vi "Save Load.vi"(6 "error in":errorcluster, 7 "save/load cluster":T3={"OK Button"=FALSE, "OK Button 2"=FALSE, "OK Button 3"=TRUE, "OK Button 4"=FALSE}, 11 "home path":path=path "C:/control") -> (4 "error out 3":errorcluster)   [LabVIEW 2016, in "Save Load.lvlib"]
doc: "Takes a vi and saves or loads set values depending on which cluster value is chosen"
uses:
  Save Load.lvlib
  Users/wymanm/Desktop/Control computer - Copy/control/control vi/ion Source/Ion Source/ion source llb.lvlib
  save or load.ctl
  all or current.ctl
  file or temp.ctl
  Users/wymanm/Desktop/Control computer - Copy/control/control vi/main/save load/saveload.ctl
  main.lvlib
  save load method.ctl
  beamline selection.ctl
panel:
  in  "Beamline Section":T1
  in  "Save Load Method":T2
  out "appended array":string[](array[string])
  out "path":path
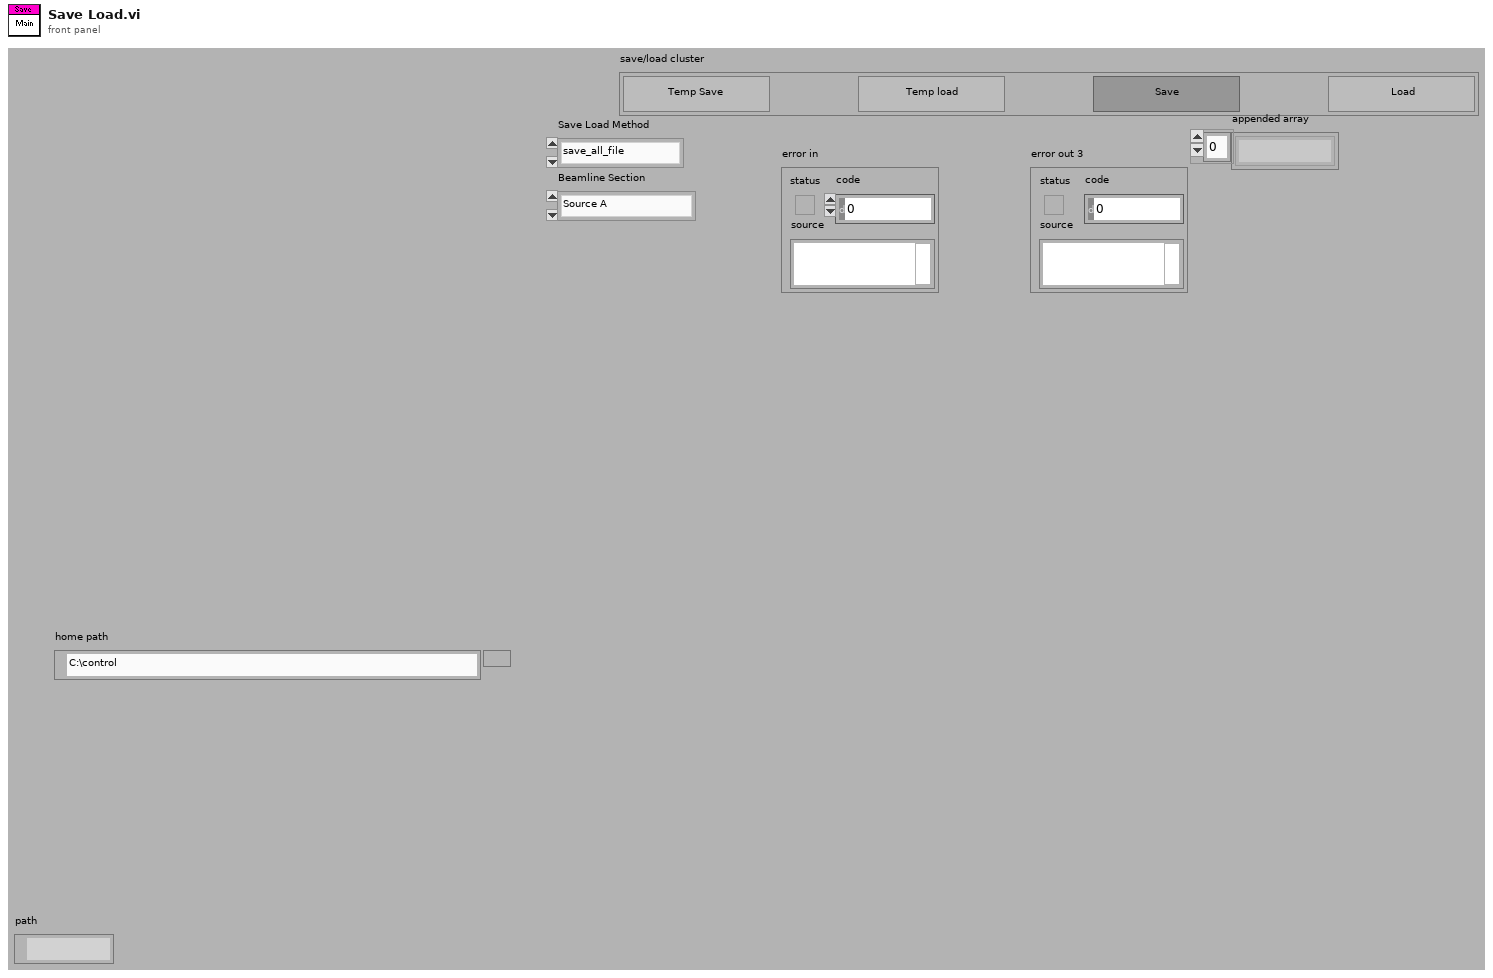
[diagram p1: front panel]
types:
  T1 = typedef "main.lvlib/beamline selection.ctl" = enum16{"Source A", "Source B", "Low Energy End", "High Energy End", "Transmission", "R30", "R45"}
  T2 = typedef "Save Load.lvlib/save load method.ctl" = enum16{"save_all_file", "save_all_temp", "save_curr_file", "save_curr_temp", "load_all_file", "load_all_temp", "load_curr_file", "load_curr_temp"}
  T3 = typedef "main.lvlib/saveload.ctl" = cluster{"OK Button":bool, "OK Button 2":bool, "OK Button 3":bool, "OK Button 4":bool}
  T4 = enum16{"open", "replace", "create", "open or create", "replace or create", "replace or create with confirmation"}
  T5 = typedef "file or temp.ctl" = enum16{"file", "temp"}
  T6 = typedef "all or current.ctl" = enum16{"current", "all"}
  T7 = typedef "save or load.ctl" = enum16{"save", "load"}
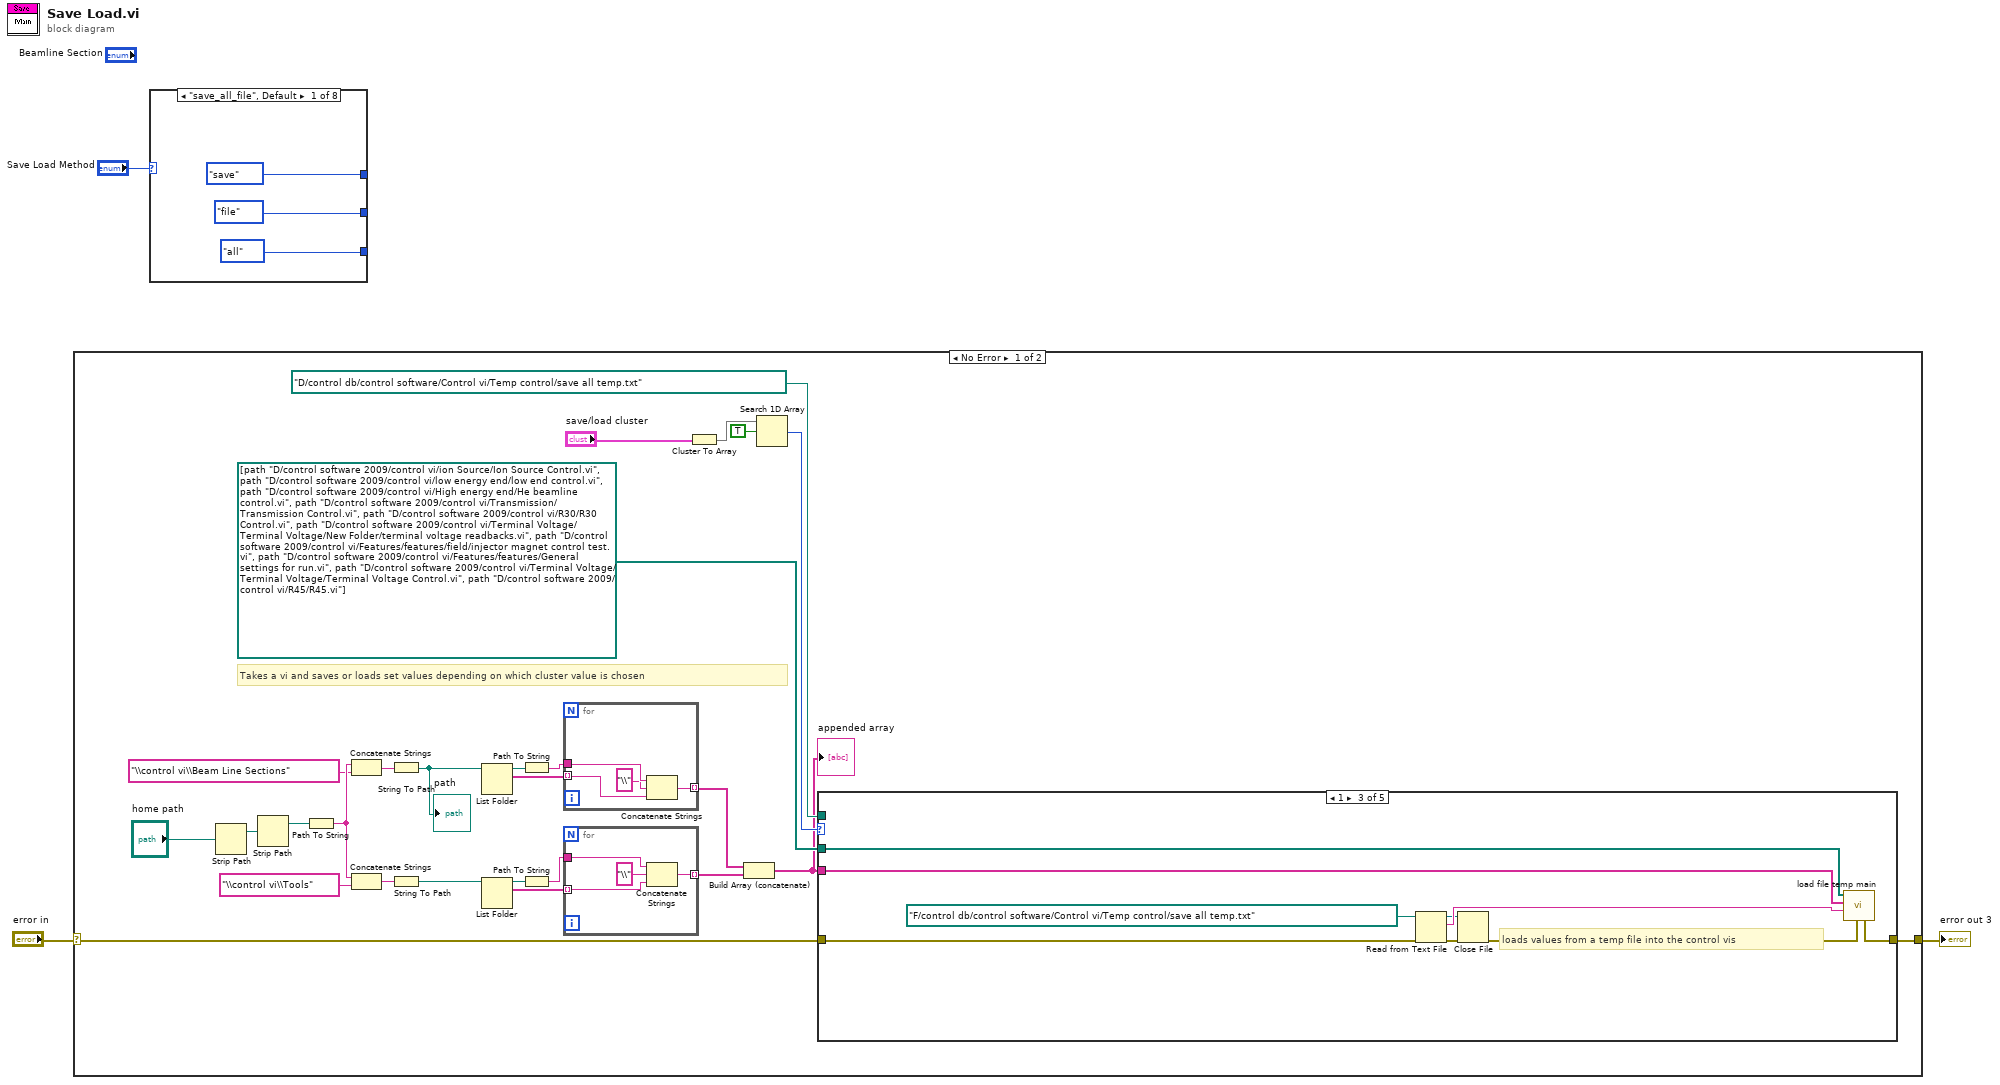
[diagram p0: block diagram]
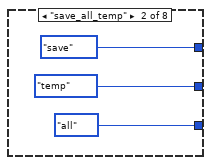
[diagram p2: hidden frame]
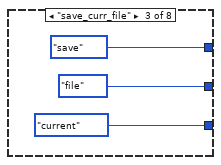
[diagram p3: hidden frame]
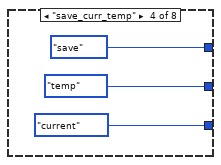
[diagram p4: hidden frame]
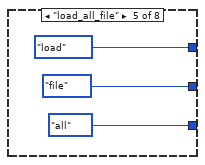
[diagram p5: hidden frame]
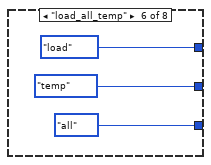
[diagram p6: hidden frame]
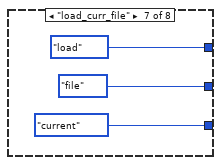
[diagram p7: hidden frame]
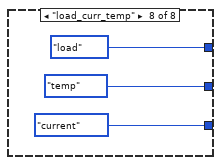
[diagram p8: hidden frame]
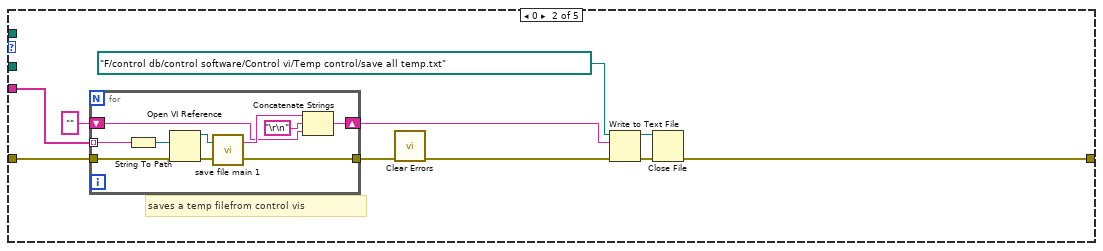
[diagram p10: hidden frame]
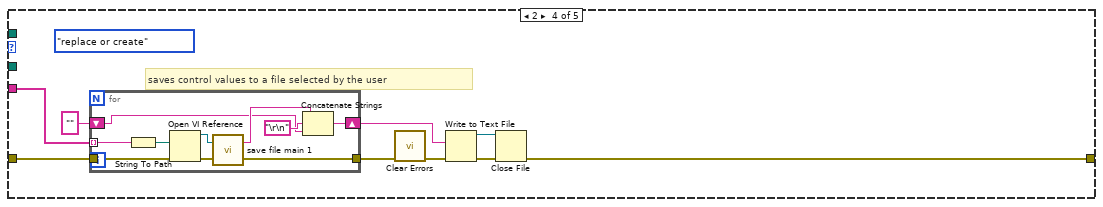
[diagram p11: hidden frame]
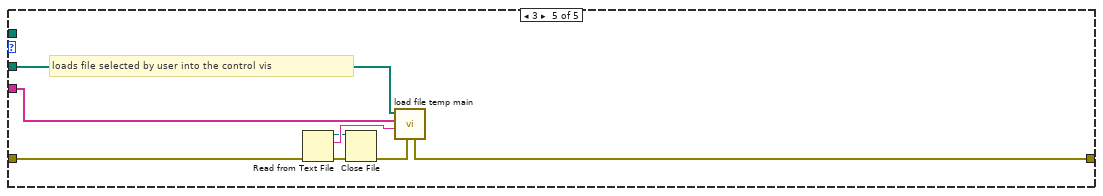
[diagram p12: hidden frame]
diagram:
  n1 = case shown="No Error" "error in" {
    selector: "error in" -> [w24 w96]
    tunnel: [w25 w96] -> w3
    frame No Error {
      # "Takes a vi and saves or loads set values depending on which cluster value is chosen"
      n2 = Strip Path(path="home path") -> (stripped path=w5:path)  [unwired: 1 out]
      n3 = Strip Path(path=w5) -> (stripped path=w4:path)  [unwired: 1 out]
      n4 = Path To String(path=w4) -> (string=w13:string)
      n5 = Concatenate Strings(w13, "\\control vi\\Beam Line Sections" ("string")) -> (w11:string)
      n6 = Concatenate Strings(w13, "\\control vi\\Tools" ("string")) -> (w14:string)
      n7 = String To Path(string=w11) -> (path=w12:path)
      "path" <- w12
      n8 = String To Path(string=w14) -> (path=w15:path)
      n9 = List Folder(path=w12) -> (path out=w21:path, filenames=w20:string[])  [unwired: 3 in, 2 out]
      n10 = List Folder(path=w15) -> (path out=w16:path, filenames=w18:string[])  [unwired: 3 in, 2 out]
      n11 = Path To String(path=w21) -> (string=w19:string)
      n12 = Path To String(path=w16) -> (string=w17:string)
      n13 = for {
        tunnel: w19 -> [w34]
        tunnel: w20 -> [w32] mode=indexing
        tunnel: [w31] -> w22 mode=indexing
        n14 = Concatenate Strings(w34, "\\" ("string"), w32) -> (w31:string)
      }
      n15 = for {
        tunnel: w17 -> [w38]
        tunnel: w18 -> [w36] mode=indexing
        tunnel: [w35] -> w23 mode=indexing
        n16 = Concatenate Strings(w38, "\\" ("string"), w36) -> (w35:string)
      }
      n17 = Cluster To Array(cluster="save/load cluster") -> (array=w29:bool[])
      n18 = Build Array (concatenate)(w22, w23) -> (w7:string[])
      "appended array" <- w7
      n19 = Search 1D Array(1D array=w29, element=TRUE) -> (index of element=w27:i32)  [unwired: 1 out]
      n20 = case shown="1" w27 {
        tunnel: path "D:/control db/control software/Control vi/Temp control/save all temp.txt" ("file path (use dialog)") -> [_ _ _ _ _]
        tunnel: path[] [path "D:/control software 2009/control vi/ion Source/Ion Source Control.vi", path "D:/control software 2009/control vi/low energy end/low end control.vi", path "D:/control software 2009/control vi/High energy end/He beamline control.vi", path "D:/control software 2009/control vi/Transmission/Transmission Control.vi", path "D:/control software 2009/control vi/R30/R30 Control.vi", path "D:/control software 2009/control vi/Terminal Voltage/Terminal Voltage/New Folder/terminal voltage readbacks.vi", path "D:/control software 2009/control vi/Features/features/field/injector magnet control test.vi", path "D:/control software 2009/control vi/Features/features/General settings for run.vi", path "D:/control software 2009/control vi/Terminal Voltage/Terminal Voltage/Terminal Voltage Control.vi", path "D:/control software 2009/control vi/R45/R45.vi"] ("Start vi array") -> [_ _ w68 _ w95]
        tunnel: w24 -> [w39 w47 w65 w76 w89]
        tunnel: [w39 w43 w64 w72 w93] -> w25
        tunnel: w7 -> [_ w40 w60 w69 w88]
        frame -1, Default {
          # "null case, does nothing"
        }
        frame 0 {
          # "saves a temp filefrom control vis"
          n21 = for {
            tunnel: [w57] -> w42
            tunnel: w47 -> [w56]
            shift-right: [w52] -> w49
            shift-left: "" -> [w53]
            tunnel: w40 -> [w51] mode=indexing
            n22 = String To Path(string=w51) -> (path=w50:path)
            n23 = Open VI Reference(vi path=w50, error in (no error)=w56) -> (vi reference=w59:refnum<vi>, error out=w58:errorcluster)  [unwired: 4 out]
            n24 = call "save file main 1.vi"("error in (no error)"=w58, "VI Refnum"=w59) -> ("error out 2"=w57:errorcluster, "String"=w54:string)
            n25 = Concatenate Strings(w54, "\r\n", w53) -> (w52:string)
          }
          n26 = call <vilib>:"Clear Errors.vi"("error in (no error)"=w42) -> ("error out"=w41:errorcluster)  [unwired: 1 in, 5 out]
          n27 = Write to Text File(file (use dialog)=path "F:/control db/control software/Control vi/Temp control/save all temp.txt" ("file path (use dialog)"), text=w49, error in=w41) -> (refnum out=w45:refnum<file>, error out=w44:errorcluster)  [unwired: 1 in, 1 out]
          n28 = Close File(refnum=w45, error in=w44) -> (error out=w43:errorcluster)  [unwired: 1 out]
        }
        frame 1 {
          # "loads values from a temp file into the control vis"
          n29 = Read from Text File(file (use dialog)=path "F:/control db/control software/Control vi/Temp control/save all temp.txt" ("file path (use dialog)"), error in=w65) -> (refnum out=w63:refnum<file>, text=w66:string, error out=w62:errorcluster)  [unwired: 3 out]
          n30 = Close File(refnum=w63, error in=w62) -> (error out=w61:errorcluster)  [unwired: 1 out]
          n31 = call "load file temp main.vi"("error in (no error)"=w61, "text"=w66, "vi array"=w60, "Start vi array"=w68) -> ("error out"=w64:errorcluster)  [unwired: 7 in]
        }
        frame 2 {
          (unwired) T4."replace or create" ("operation (0:open)")
          # "saves control values to a file selected by the user"
          n32 = for {
            tunnel: [w85] -> w71
            tunnel: w76 -> [w84]
            shift-right: [w80] -> w77
            shift-left: "" -> [w81]
            tunnel: w69 -> [w79] mode=indexing
            n33 = String To Path(string=w79) -> (path=w78:path)
            n34 = Open VI Reference(vi path=w78, error in (no error)=w84) -> (vi reference=w87:refnum<vi>, error out=w86:errorcluster)  [unwired: 4 out]
            n35 = call "save file main 1.vi"("error in (no error)"=w86, "VI Refnum"=w87) -> ("error out 2"=w85:errorcluster, "String"=w82:string)
            n36 = Concatenate Strings(w82, "\r\n", w81) -> (w80:string)
          }
          n37 = call <vilib>:"Clear Errors.vi"("error in (no error)"=w71) -> ("error out"=w70:errorcluster)  [unwired: 1 in, 5 out]
          n38 = Write to Text File(text=w77, error in=w70) -> (refnum out=w74:refnum<file>, error out=w73:errorcluster)  [unwired: 1 in, 2 out]
          n39 = Close File(refnum=w74, error in=w73) -> (error out=w72:errorcluster)  [unwired: 1 out]
        }
        frame 3 {
          # "loads file selected by user into the control vis"
          n40 = Read from Text File(error in=w89) -> (refnum out=w91:refnum<file>, text=w94:string, error out=w92:errorcluster)  [unwired: 4 out]
          n41 = Close File(refnum=w91, error in=w92) -> (error out=w90:errorcluster)  [unwired: 1 out]
          n42 = call "load file temp main.vi"("error in (no error)"=w90, "text"=w94, "vi array"=w88, "Start vi array"=w95) -> ("error out"=w93:errorcluster)  [unwired: 7 in]
        }
      }
    }
    frame Error {
    }
  }
  "error out 3" <- w3
  n43 = case shown="\"save_all_file\", Default" "Save Load Method" {
    tunnel: [save_or_load."save" save_or_load."save" save_or_load."save" save_or_load."save" save_or_load."load" save_or_load."load" save_or_load."load" save_or_load."load"] -> _
    tunnel: [all_or_current."all" all_or_current."all" all_or_current."current" all_or_current."current" all_or_current."all" all_or_current."all" all_or_current."current" all_or_current."current"] -> _
    tunnel: [file_or_temp."file" file_or_temp."temp" file_or_temp."file" file_or_temp."temp" file_or_temp."file" file_or_temp."temp" file_or_temp."file" file_or_temp."temp"] -> _
    frame "save_all_file", Default {
    }
    frame "save_all_temp" {
    }
    frame "save_curr_file" {
    }
    frame "save_curr_temp" {
    }
    frame "load_all_file" {
    }
    frame "load_all_temp" {
    }
    frame "load_curr_file" {
    }
    frame "load_curr_temp" {
    }
  }
